vi "Receive Event.vi"(8 "Error In":errorcluster, 9 "Event Data":refnum<class "Event Data.lvclass">, 10 "Event Name":string, 11 "Event Receiver In":refnum<class "Event Receiver.lvclass">) -> (0 "Error Out":errorcluster, 3 "Event Receiver Out":refnum<class "Event Receiver.lvclass">)   [LabVIEW 2021, in "EventSourceActor.lvlib" / "Event Receiver.lvlib" / "Event Receiver.lvclass"]
uses:
  Event Receiver.lvclass
  Template Source/Event Data/Event Data.lvclass
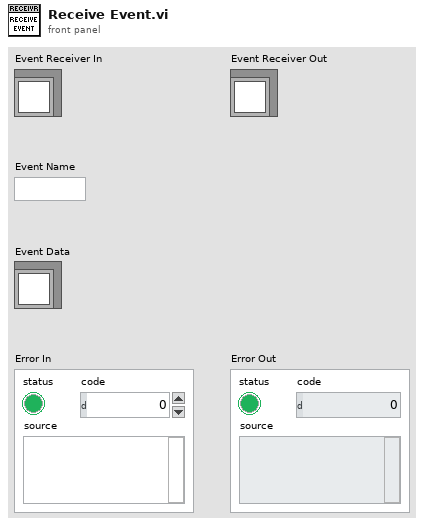
[diagram p1: front panel]
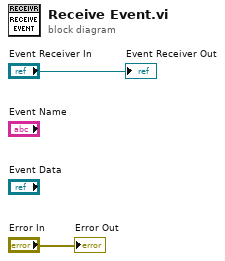
[diagram p0: block diagram]
diagram:
  "Event Receiver Out" <- "Event Receiver In"
  "Error Out" <- "Error In"
